vi "Servo Ignore if not initialized.vi"(11 "Command in":T1) -> (3 "command out":T1)   [LabVIEW 2017, in "Servo drive module.lvlib"]
doc: "Returns enum with command to ignore message, if module is not initialized. In that case, only \"initialize\" command will be accepted."
uses:
  Servo drive module.lvlib
  ctl/Servo commands.ctl
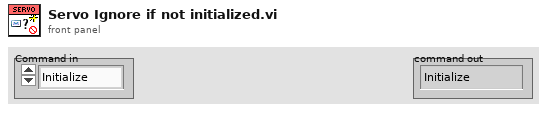
[diagram p1: front panel]
types:
  T1 = typedef "Servo drive module.lvlib/Servo commands.ctl" = enum16{"Initialize", "Update", "Move by", "Move to", "Stop", "Ignore", "End"}
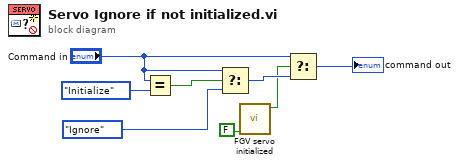
[diagram p0: block diagram]
diagram:
  n1 = Equal?(x="Command in", y=Servo_commands."Initialize") -> (x = y?=w5:bool)
  n2 = Select(t="Command in", s=w5, f=Servo_commands."Ignore" ("y")) -> (s? t:f=w8:T1)
  n3 = call "FGV servo initialized.vi"("Write?(F)"=FALSE) -> ("Initialized out"=w1:bool)  [unwired: 10 in]
  n4 = Select(t="Command in", s=w1, f=w8) -> (s? t:f=→"command out":T1)
